vi "Set (Strings).vi"(5 "Tags":string[](array[string]), 7 "error in (no error)":errorcluster, 9 "Values":string[](array[string]), 10 "ByRef Variant Repsitory in":refnum<data-value>) -> (0 "error out":errorcluster)   [LabVIEW 2015, in "ByRef Variant Repository.lvlib"]
uses:
  ByRef Variant Repository.lvlib
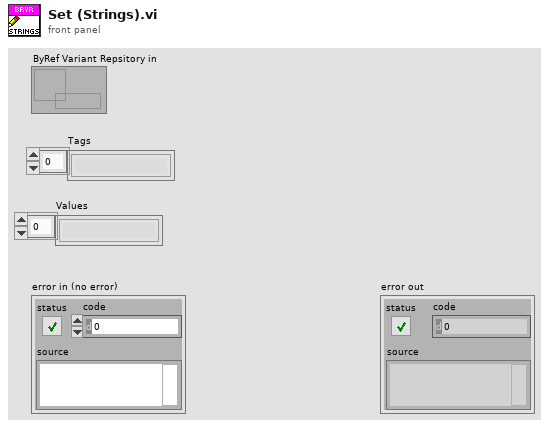
[diagram p1: front panel]
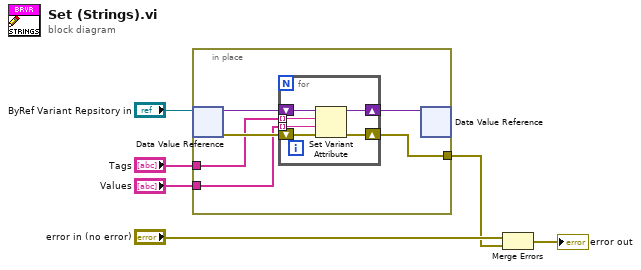
[diagram p0: block diagram]
diagram:
  n1 = in-place {
    in-place-border: [w9] -> w4
    in-place-border: "Tags" -> [w8]
    in-place-border: "Values" -> [w7]
    n2 = in-place-dvr #1("ByRef Variant Repsitory in") -> (w11:variant, w12:errorcluster)
    n3 = for {
      tunnel: w8 -> [w14] mode=indexing
      shift-right: [w15] -> w9
      shift-left: w12 -> [w18]
      shift-right: [w16] -> w10
      shift-left: w11 -> [w17]
      tunnel: w7 -> [w13] mode=indexing
      n4 = Set Variant Attribute(Variant=w17, name=w14, value=w13, error in=w18) -> (Variant out=w16:variant, error out=w15:errorcluster)  [unwired: 1 out]
    }
    n5 = in-place-dvr #1(w10) -> ()  [unwired: 2 out]
  }
  n6 = Merge Errors("error in (no error)", w4) -> (→"error out":errorcluster)
